vi "CTI.vi"(0 "System no.":i32=1 min=1 max=4 step=1, 2 "TriggerIn to set":string[](array[string]), 4 "No.of digits":i16=4, 5 "error in":errorcluster, 6 "CTI parameter ID":i32[](array[numeric]), 10 "Parameter value":string[](array[string])) -> (14 "Controller error":bool, 19 "error out":errorcluster)   [LabVIEW 2020]
doc: "This VI configures the Trigger Input conditions for the given digital input line, waits 100 ms and queries ERR?. The trigger input actions only become active when enabled with TRI. See user manual for available CTI Parameter IDs, parameter numbers and values. No. of digits is the number of digits after the decimal point in the numeric parameter value(s) that will be sent. Controller error is TRUE if selected system reports error code which is not 0. \n\nE-709:"
panel:
  # "This vi configures the Trigger Input conditions for the given digital input line, waits\n100 ms and queries ERR?. The trigger input actions only become active when enabled \nwith TRI."
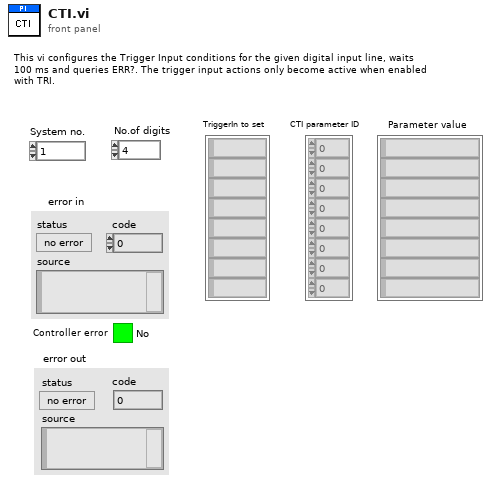
[diagram p1: front panel]
types:
  T1 = enum16{"Disable error check", "Force error check", "Use global settings"}
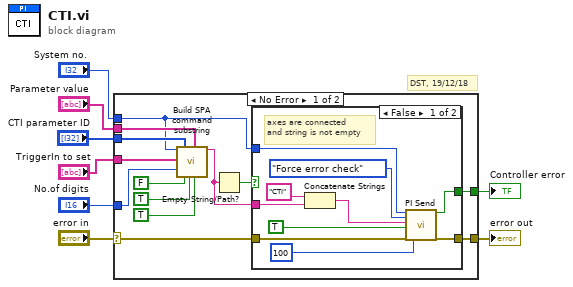
[diagram p0: block diagram]
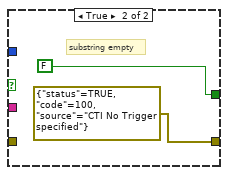
[diagram p2: hidden frame]
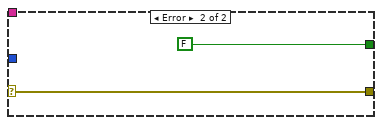
[diagram p3: hidden frame]
diagram:
  # "DST, 19/12/18"
  n1 = case shown="No Error" "error in" {
    selector: "error in" -> [w11 w34]
    tunnel: [w21 w34] -> w8
    tunnel: "No.of digits" -> [w20 _]
    tunnel: "System no." -> [w16 _]
    tunnel: "TriggerIn to set" -> [w19 _]
    tunnel: "CTI parameter ID" -> [w18 _]
    tunnel: "Parameter value" -> [w17 _]
    tunnel: [w12 FALSE ("Controller error")] -> w2
    frame No Error {
      n2 = call "Build SPA command substring.vi"("System no."=w16, "Axes to set"=w19, "No. of digits"=w20, "Parameter number"=w18, "Parameter no. format \n(Decimal: FALSE)"=FALSE ("Parameter no. format \n(Decimal: FALSE)"), "Parameter format \n(Num.: FALSE)"=TRUE ("Parameter format \n(Num.: FALSE)"), "Parameter strings"=w17, "With space?"=TRUE) -> ("SPA command substring"=w10:string)  [unwired: 2 in, 9 out]
      n3 = Empty String/Path?(string/path=w10) -> (empty?=w9:bool)
      n4 = case shown="False" w9 {
        tunnel: w10 -> [w30 _]
        tunnel: [w23 errorcluster {"status"=TRUE, "code"=100, "source"="CTI No Trigger specified"} ("error out")] -> w21
        tunnel: w11 -> [w27 _]
        tunnel: w16 -> [w26 _]
        tunnel: [w22 FALSE ("Controller error")] -> w12
        frame False {
          # "axes are connected \nand string is not empty"
          n5 = Concatenate Strings("CTI", w30) -> (w28:string)
          n6 = call "PI Send.vi"("System no."=w26, "Error check settings"=T1."Force error check", "String to send"=w28, "Attach termination char.?"=TRUE ("Attach Linefeed?"), "error in"=w27, "Delay before error check (ms)"=u32 100 ("milliseconds to wait")) -> ("Controller error"=w22:bool, "error out"=w23:errorcluster)  [unwired: 12 out]
        }
        frame True {
          # "substring empty"
        }
      }
    }
    frame Error {
    }
  }
  "error out" <- w8
  "Controller error" <- w2
